vi "Grab.vi"(8 "error in (no error)":errorcluster, 10 "Image in":T1, 11 "IMAQdx Camera in":refnum<class "IMAQdx Camera.lvclass">) -> (0 "error out":errorcluster, 2 "Image out":T1, 3 "IMAQdx Camera out":refnum<class "IMAQdx Camera.lvclass">)   [LabVIEW 2011, in "IMAQdx Camera.lvclass"]
uses:
  IMAQdx Camera.lvclass
  <vilib>/vision/Image Controls.llb/IMAQ Image.ctl
  IMAQdx Camera.lvclass/IMAQdx Camera.ctl
  <vilib>/vision/driver/NI_Vision_Acquisition_Software.lvlib
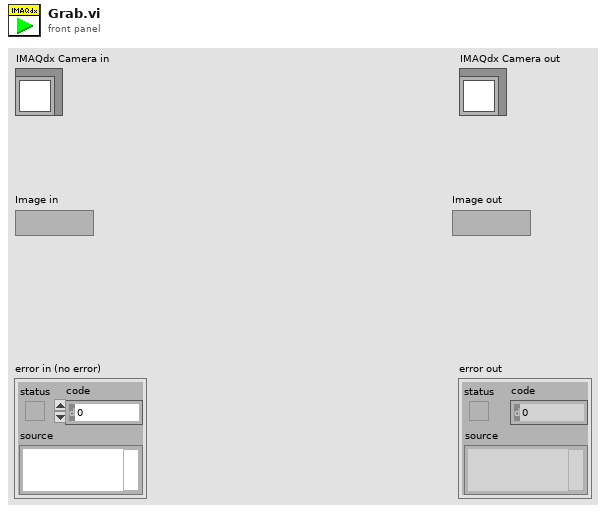
[diagram p1: front panel]
types:
  T1 = typedef "IMAQ Image.ctl" = refnum<image>
  T2 = typedef "IMAQdx.ctl" = refnum<k21>
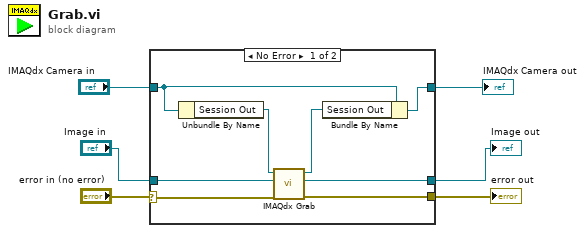
[diagram p0: block diagram]
diagram:
  n1 = case shown="No Error" "error in (no error)" {
    selector: "error in (no error)" -> [w7 w16]
    tunnel: [w14 w16] -> w6
    tunnel: [w13 w15] -> w5
    tunnel: "Image in" -> [w12 w15]
    tunnel: "IMAQdx Camera in" -> [w9 w17]
    tunnel: [w8 w17] -> w2
    frame No Error {
      n2 = Unbundle By Name(w9) -> ("Session Out"=w11:T2)
      n3 = call <vilib>:"IMAQdx Grab.vi"("error in"=w7, "Image In"=w12, "Session In"=w11) -> ("error out"=w14:errorcluster, "Image Out"=w13:T1, "Session Out"=w10:T2)  [unwired: 5 in, 1 out]
      n4 = Bundle By Name(cluster=w9, "Session Out"=w10) -> (w8:refnum<class "IMAQdx Camera.lvclass">)
    }
    frame Error {
    }
  }
  "error out" <- w6
  "IMAQdx Camera out" <- w2
  "Image out" <- w5
